vi "Set Voltage Copy.vi"(8 "error in (no error)":errorcluster, 9 "voltage copy (off)":bool, 10 "Channel (0: Channel 1)":T1 items=["Channel 1", "Channel 2"], 11 "VISA resource name":refnum<visa-resource-name>) -> (0 "error out":errorcluster, 3 "VISA resource name out":refnum<visa-resource-name>)   [LabVIEW 2009, in "Tektronix AFG 3000 Series.lvlib"]
doc: "Allows you to copy the voltage level of one channel to another channel. The channel specified in the command is copied to the other channel, and the other channel's voltage levels mirror the original until copying is turned off."
uses:
  Tektronix AFG 3000 Series.lvlib
  controls.llb/Channel.ctl
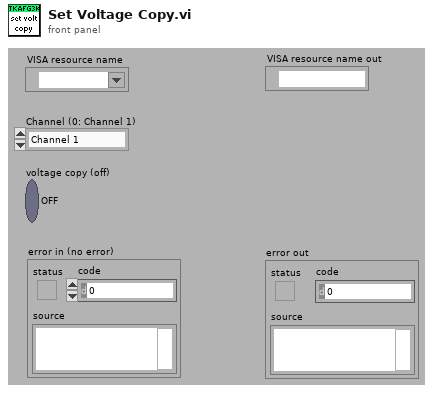
[diagram p1: front panel]
types:
  T1 = typedef "Channel.ctl" = u16
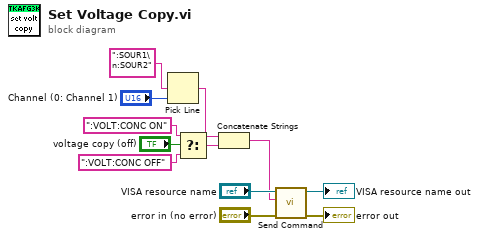
[diagram p0: block diagram]
diagram:
  n1 = Pick Line(multi-line string=":SOUR1\n:SOUR2", line index="Channel (0: Channel 1)") -> (output string=w4:string)  [unwired: 1 out]
  n2 = Select(t=":VOLT:CONC ON" ("multi-line string"), s="voltage copy (off)", f=":VOLT:CONC OFF" ("multi-line string")) -> (s? t:f=w2:string)
  n3 = Concatenate Strings(w4, w2) -> (w1:string)
  n4 = call "Send Command.vi"("error in (no error)"="error in (no error)", "write buffer"=w1, "VISA resource name"="VISA resource name") -> ("error out"=→"error out":errorcluster, "VISA resource name out"=→"VISA resource name out":refnum<visa-resource-name>)  [unwired: 7 out]
